vi "Dequeue Message.vi"(8 "error in (no error)":T1 caption="entrée d'erreur (pas d'erreur)", 11 "File d'attente de messages":refnum<queue>) -> (0 "error out":T1 caption="sortie d'erreur", 1 "Données de message":variant, 2 "Message":string, 3 "File d'attente de message dup.":refnum<queue>)   [LabVIEW 2012, in "Message Queue.lvlib"]
doc: "Ce VI extrait des messages de la file d'attente de messages. Il dispose d'une gestion particulière des erreurs pour gérer les erreurs survenant à la dernière itération de la boucle de gestion de messages.\n\nPas d'erreur: fonctionnement normal de supprimer le premier élément d'une file d'attente.\nErreur : vérifier si c'est un code d'erreur à ignorer. Dans ce cas, effacer l'erreur et supprimer le premier élément d'une file d'attente normalement. Sinon, renvoyer l'erreur et mettre un message 'Arrêter' dans la file d'attente de messages."
uses:
  Message Queue.lvlib
  Message Cluster.ctl
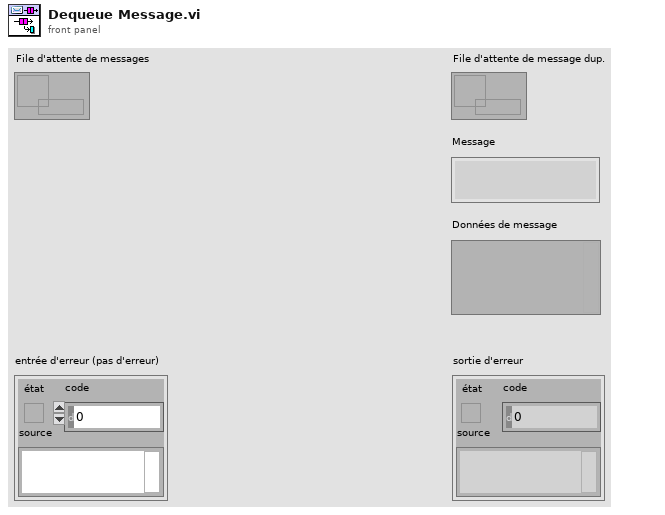
[diagram p1: front panel]
types:
  T1 = cluster{"état":bool, "code":i32, "source":string}
  T2 = typedef "Message Queue.lvlib/Message Cluster.ctl" = cluster{"Message":string, "Données de message":variant}
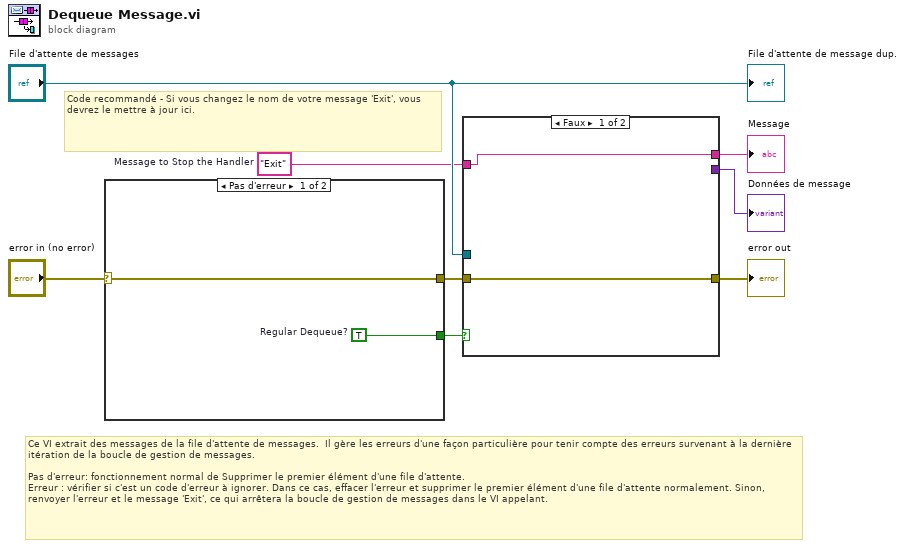
[diagram p0: block diagram]
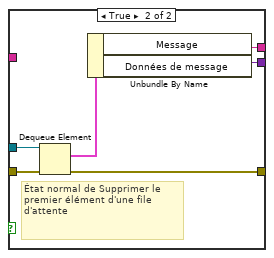
[diagram p2: hidden frame]
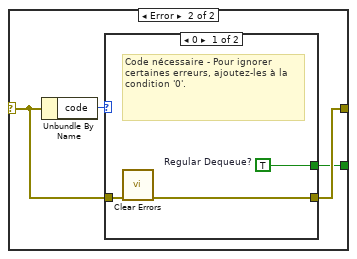
[diagram p3: hidden frame]
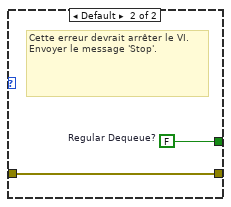
[diagram p4: hidden frame]
diagram:
  w1 = "Exit"  # Message to Stop the Handler
  # "Code recommandé - Si vous changez le nom de votre message 'Exit', vous devrez le mettre à jour ici."
  # "Ce VI extrait des messages de la file d'attente de messages.  Il gère les erreurs d'une façon particulière pour tenir compte des erreurs survenant à la dernière itération de la boucle de gestion de messages.\n\nPas d'erreur: fonctionnement normal de Supprimer le premier élément d'une file d'attente.\nErreur : vérifier si c'est un code d'erreur à ignorer. Dans ce cas, effacer l'erreur et supprimer le premier élément d'une file d'attente normalement. Sinon, renvoyer l'erreur et le message 'Exit', ce qui arrêtera la boucle de gestion de messages dans le VI appelant."
  n1 = case shown="Pas d'erreur" "error in (no error)" {
    selector: "error in (no error)" -> [w10 w13]
    tunnel: [w10 w12] -> w6
    tunnel: [w9 w11] -> w5
    frame No Error {
      w9 = TRUE  # Regular Dequeue?
    }
    frame Error {
      n2 = Unbundle By Name(w13) -> ("code"=w14:i32)
      n3 = case shown="0" w14 {
        tunnel: [w17 w19] -> w12
        tunnel: w13 -> [w16 w19]
        tunnel: [w15 w18] -> w11
        frame 0 {
          w15 = TRUE  # Regular Dequeue?
          # "Code nécessaire - Pour ignorer certaines erreurs, ajoutez-les à la condition '0'."
          n4 = call <vilib>:"Clear Errors.vi"("error in (no error)"=w16) -> ("error out"=w17:errorcluster)  [unwired: 6 in]
        }
        frame Default {
          w18 = FALSE  # Regular Dequeue?
          # "Cette erreur devrait arrêter le VI. Envoyer le message 'Stop'."
        }
      }
    }
  }
  n5 = case shown="Faux" w5 {
    tunnel: [w21 w27] -> w7
    tunnel: w6 -> [w21 w26]
    tunnel: "File d'attente de messages" -> [_ w25]
    tunnel: [w20 w23] -> w3
    tunnel: [_ w22] -> w2
    tunnel: w1 -> [w20 _]
    frame False {
    }
    frame True {
      # "État normal de Supprimer le premier élément d'une file d'attente"
      n6 = Dequeue Element(queue=w25, error in (no error)=w26) -> (element=w24:T2, error out=w27:errorcluster)  [unwired: 1 in, 2 out]
      n7 = Unbundle By Name(w24) -> ("Message"=w23:string, "Données de message"=w22:variant)
    }
  }
  "error out" <- w7
  "Message" <- w3
  "Données de message" <- w2
  "File d'attente de message dup." <- "File d'attente de messages"
